vi "Write configuration.vi"(8 "error in":errorcluster, 10 "configuration":refnum<class "NISE_CEF_serializable configuration.lvclass">, 11 "Cfg Channel in":refnum<class "channel node.lvclass">) -> (0 "error out":errorcluster, 3 "Cfg Channel out":refnum<class "channel node.lvclass">)   [LabVIEW 2013, in "channel node.lvclass"]
uses:
  channel node.lvclass
  Configuration Framework/serializable configuration/NISE_CEF_serializable configuration.lvclass
  channel configuration/channel configuration.lvclass
  channel node.lvclass/channel node.ctl
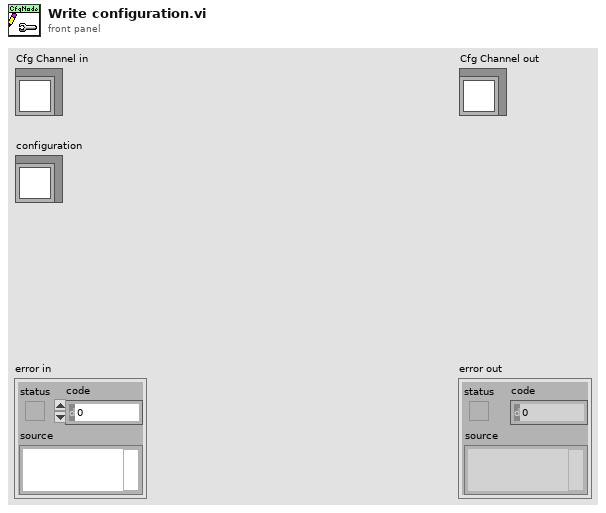
[diagram p1: front panel]
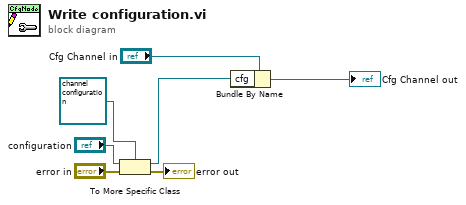
[diagram p0: block diagram]
diagram:
  n1 = To More Specific Class(target class=refnum<class "channel configuration.lvclass"> refnum ("channel config object.lvclass"), reference="configuration", error in="error in") -> (specific class reference=w2:refnum<class "channel configuration.lvclass">, error out=→"error out":errorcluster)
  n2 = Bundle By Name(cluster="Cfg Channel in", "cfg"=w2) -> (→"Cfg Channel out":refnum<class "channel node.lvclass">)
